vi "Add Data Byte.vi"(6 "Byte order":T1, 8 "error in (no error)":errorcluster, 9 "Data":u8, 10 "Action":T2, 11 "I2C waveform info":T3) -> (0 "error out":errorcluster, 3 "I2C waveform info out":T3)   [LabVIEW 2009, in "IDW.lvlib"]
doc: "Adds a data byte to the I2C waveform. \n\nEach bit of the byte is added in the <b>Byte order</b> order. For a <b>Receive (Rx)</b> action, the SDA line is released and a single sample in the center of the clock pulse is compared against the expected value. For a <b>Transmit (Tx)</b> action, the value is written to the SDA line according to the timing parameters specified by the <b>Init</b> VI.\n\nTiming parameters that affect this waveform segment's length are: <b>tSU;DAT</b>, <b>tHIGH</b>, and <b>tHD;DAT</b>."
uses:
  IDW.lvlib
  _Typedefs/Waveform info.ctl
  _Typedefs/Timing - ticks.ctl
  _Typedefs/Default transition action.ctl
  _Typedefs/Bit type.ctl
  _Typedefs/Bus operation.ctl
  _Typedefs/Byte order.ctl
  _Polymorphics/Interpret Data - Byte.vi
  _Typedefs/Transition action.ctl
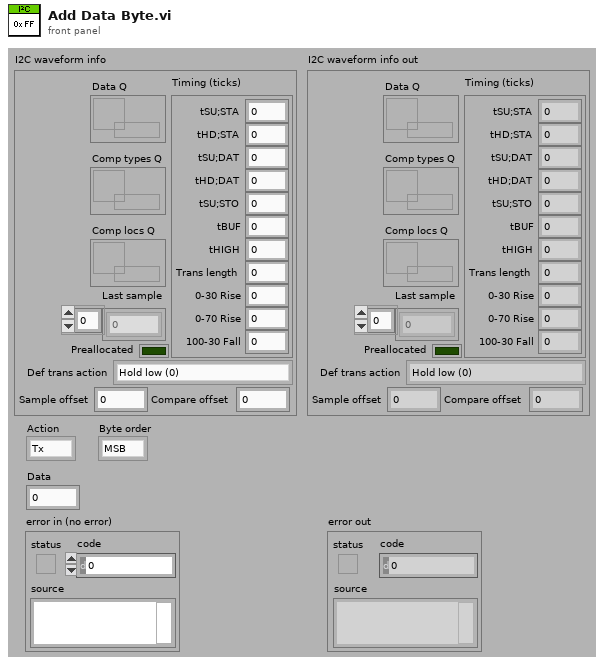
[diagram p1: front panel]
types:
  T1 = typedef "IDW.lvlib/Byte order.ctl" = enum16{"MSB", "LSB"}
  T2 = typedef "IDW.lvlib/Bus operation.ctl" = enum16{"Tx", "Rx"}
  T3 = typedef "IDW.lvlib/Waveform info.ctl" = cluster{"Last sample":u8[], "Sample offset":u64, "Compare offset":u64, "Timing (ticks)":T4, "Preallocated":bool, "Def trans action":T5, "Data Q":refnum<queue>, "Comp types Q":refnum<queue>, "Comp locs Q":refnum<queue>}
  T4 = typedef "IDW.lvlib/Timing - ticks.ctl" = cluster{"tSU;STA":i32, "tHD;STA":i32, "tSU;DAT":i32, "tHD;DAT":i32, "tSU;STO":i32, "tBUF":i32, "tHIGH":i32, "Trans length":i32, "0-30 Rise":i32, "0-70 Rise":i32, "100-30 Fall":i32}
  T5 = typedef "IDW.lvlib/Default transition action.ctl" = enum16{"Hold low (0)", "Release (Z)", "Set up next value", "Hold previous value", "Preserve tHD;DAT and tSU;DAT"}
  T6 = typedef "IDW.lvlib/Transition action.ctl" = enum16{"Hold low (0)", "Release (Z)", "Set up next value", "Hold previous value", "Preserve tHD;DAT and tSU;DAT", "<Use session default>"}
  T7 = typedef "IDW.lvlib/Bit type.ctl" = enum16{"ACK", "Data"}
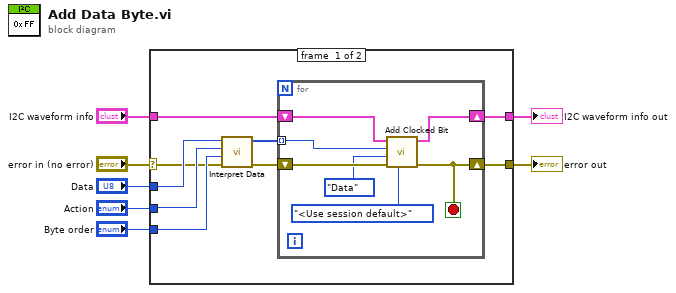
[diagram p0: block diagram]
diagram:
  n1 = case shown="No Error" "error in (no error)" {
    selector: "error in (no error)" -> [w8 w25]
    tunnel: "Action" -> [w10 _]
    tunnel: "Data" -> [w13 _]
    tunnel: [w16 w24] -> w5
    tunnel: "I2C waveform info" -> [w15 w24]
    tunnel: "Byte order" -> [w11 _]
    tunnel: [w14 w25] -> w1
    frame #0 {
      n2 = call-poly "Interpret Data.vi"("error in (no error)"=w8, "Byte order"=w11, "Action"=w10, "Data"=w13) -> ("error out"=w9:errorcluster, "Digital data bits"=w12:u8[])  [unwired: 6 out]
      n3 = for {
        shift-right: [w22] -> w16
        shift-left: w15 -> [w23]
        tunnel: w12 -> [w21] mode=indexing
        shift-right: [w19] -> w14
        shift-left: w9 -> [w20]
        stop <- w19 stop-if-true
        n4 = call "Add Clocked Bit.vi"("Transition action"=Transition_action."<Use session default>", "error in (no error)"=w20, "Bit type"=Bit_type."Data", "Bit value"=w21, "I2C waveform info"=w23) -> ("error out"=w19:errorcluster, "I2C waveform info out"=w22:T3)  [unwired: 5 out]
      }
    }
    frame #1 {
    }
  }
  "I2C waveform info out" <- w5
  "error out" <- w1
